vi "Destroy Message Queue.vi"(8 "Error In":errorcluster) -> (0 "Error Out":errorcluster)   [LabVIEW 2023, in "QSM - Main.lvlib"]
doc: "This VI destroys the message queue for the Queued State Machine template."
uses:
  QSM - Main.lvlib
  Controls/Message Queue Reference Functional Global Variable Operation.ctl
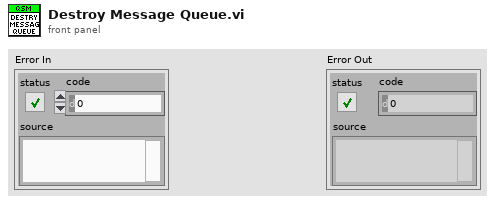
[diagram p1: front panel]
types:
  T1 = typedef "QSM - Main.lvlib/Message Queue Reference Functional Global Variable Operation.ctl" = enum16{"Set", "Get"}
  T2 = typedef "QSM - Library.lvlib/Message Queue Reference.ctl" = refnum<queue>
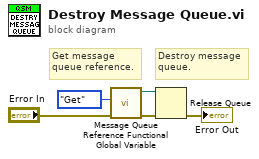
[diagram p0: block diagram]
diagram:
  # "Destroy message\nqueue."
  # "Get message\nqueue reference."
  n1 = call "Message Queue Reference Functional Global Variable.vi"("Error In"="Error In", "Operation"=Message_Queue_Reference_Functional_Global_Variable_Operation."Get") -> ("Error Out"=w4:errorcluster, "Message Queue Reference Out"=w2:T2)  [unwired: 8 in]
  n2 = Release Queue(queue=w2, error in (no error)=w4) -> (error out=→"Error Out":errorcluster)  [unwired: 1 in, 2 out]
